vi "InterceptBallSkill_Init.vi"(0 "object in":refnum<class "InterceptBallSkill.lvclass">, 5 "error in (no error)":errorcluster) -> (14 "object out":refnum<class "InterceptBallSkill.lvclass">, 19 "error out":errorcluster)   [LabVIEW 2023, in "InterceptBallSkill.lvclass"]
uses:
  InterceptBallSkill.lvclass
  C:/Users/ebert/Documents/codes/SSL/repo/SSL_AI/GoToSkill_v2_class/GoToSkill_v2.lvclass
  InterceptBallSkill.lvclass/InterceptBallSkill.ctl
  GoToSkill_v2_class/GoToSkill_v2.lvclass
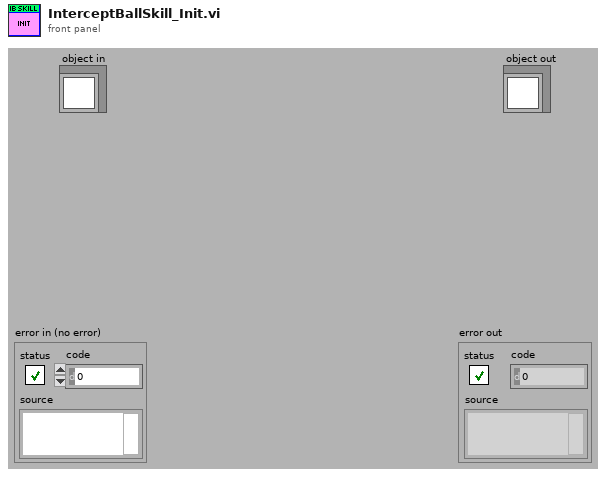
[diagram p1: front panel]
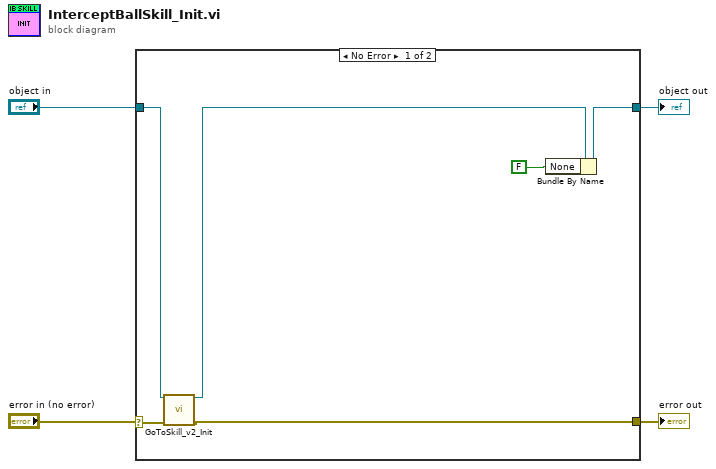
[diagram p0: block diagram]
diagram:
  n1 = case shown="No Error" "error in (no error)" {
    selector: "error in (no error)" -> [w6 w11]
    tunnel: [w10 w12] -> w4
    tunnel: "object in" -> [w8 w12]
    tunnel: [w5 w11] -> w1
    frame No Error {
      n2 = call "GoToSkill_v2_Init.vi"("object in"=w8, "error in (no error)"=w6) -> ("object out"=w7:refnum<class "InterceptBallSkill.lvclass">, "error out"=w5:errorcluster)  [unwired: 16 in]
      n3 = Bundle By Name(cluster=w7, "None"=FALSE) -> (w10:refnum<class "InterceptBallSkill.lvclass">)
    }
    frame Error {
    }
  }
  "object out" <- w4
  "error out" <- w1
